vi "Global Queue.vi"(1 "Global in":refnum<k1>) -> (0 "Global":refnum<queue>)   [LabVIEW 2018, in "Shared.lvlib"]
uses:
  Shared.lvlib
  Controls/Global.ctl
panel:
  in  "FALSE":bool
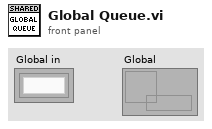
[diagram p1: front panel]
types:
  T1 = cluster{"ID":i32, "Name":string, "Parent":i32, "Queue":refnum<queue>, "Ini Path":path, "Ini Section":string, "VI Name":string, "VI Path":path, "VI Refnum":refnum<vi>, "Group":string}[]
  T2 = typedef "Shared.lvlib/Global.ctl" = cluster{"ID":i32, "Name":string, "Parent":i32, "Queue":refnum<queue>, "Ini Path":path, "Ini Section":string, "VI Name":string, "VI Path":path, "VI Refnum":refnum<vi>, "Group":string}
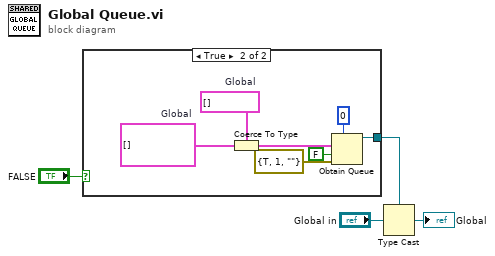
[diagram p0: block diagram]
diagram:
  n1 = case shown="True" "FALSE" {
    tunnel: [_ w11] -> w2
    frame False {
    }
    frame True {
      w6 = T1 []  # Global
      w8 = T2[] []  # Global
      n2 = Coerce To Type(0:w8, 1:w6) -> (2:w7:T1)
      n3 = Obtain Queue(max queue size (-1, unlimited)=0, element data type=w7, create if not found? (T)=FALSE, error in (no error)=errorcluster {"status"=TRUE, "code"=1, "source"=""}) -> (queue out=w11:refnum<queue>)  [unwired: 1 in, 2 out]
    }
  }
  n4 = Type Cast(type=w2, x="Global in") -> (*(type *) &x=→"Global":refnum<queue>)
